vi "mining search for scenario.vi"(6 "User":T3, 7 "Header In":string, 8 "error in (no error)":errorcluster, 10 "GET (empty)":T1, 11 "Connection Refnum":T2) -> (0 "error out":errorcluster, 1 "Template Keys":T1, 2 "Template":string, 3 "Connection Refnum":T2, 5 "new Header":string)   [LabVIEW 2011]
uses:
  server/database/Users/User Record.ctl
  Addons/internet/utils/keyedarr.llb/Keyed Array.ctl
  SI.LIB/ODBC/SQL Controls/Connection Refnum.ctl
  Addons/internet/utils/strutil.llb/Case Matching.ctl
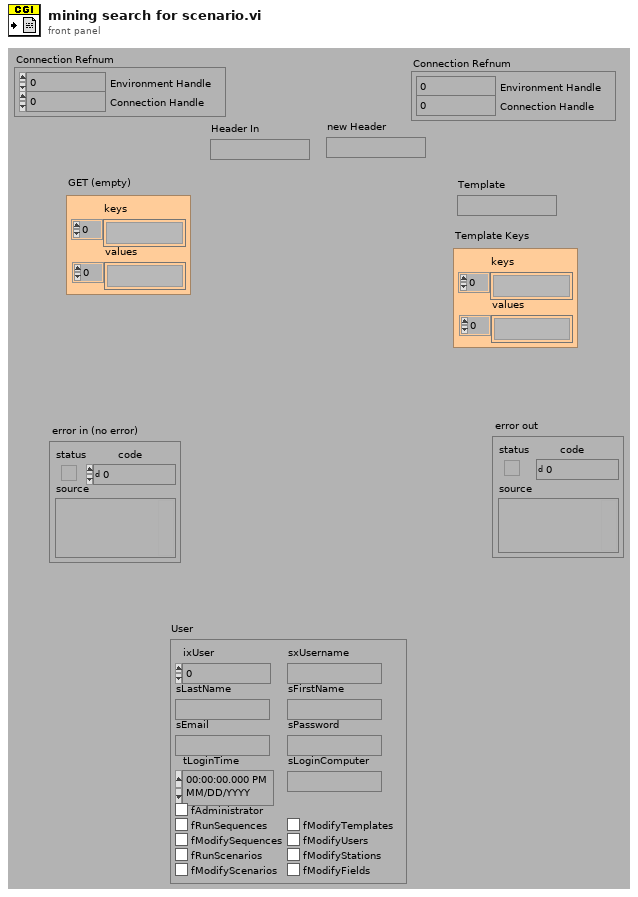
[diagram p1: front panel]
types:
  T1 = typedef "Keyed Array.ctl" = cluster{"keys":string[], "values":string[]}
  T2 = typedef "Connection Refnum.ctl" = cluster{"Environment Handle":i32, "Connection Handle":i32}
  T3 = typedef "User Record.ctl" = cluster{"ixUser":i32, "sxUsername":string, "sLastName":string, "sFirstName":string, "sEmail":string, "sPassword":string, "tLoginTime":timestamp, "sLoginComputer":string, "fAdministrator":bool, "fRunSequences":bool, "fModifySequences":bool, "fRunScenarios":bool, "fModifyScenarios":bool, "fModifyTemplates":bool, "fModifyUsers":bool, "fModifyStations":bool, "fModifyFields":bool}
  T4 = typedef "Case Matching.ctl" = enum16{"a != A", "a == A", "system"}
  T5 = typedef "Scenario Record.ctl" = cluster{"ixScenario":i32, "tCreated":timestamp, "tModified":timestamp, "sxUsername":string, "sModifiedBy":string, "sxScenarioId":string, "sDescription":string, "sLogic":string, "sResultFieldsCSV":string, "sTemplatesCSV":string, "fAutoRunReports":bool, "fSortByTemplates":bool, "fCombinePDF":bool, "Conditions":T6[]}
  T6 = typedef "Condition Record.ctl" = cluster{"iConditionIndex":i32, "sxFieldId":string, "nOperator":T7, "sMatchValue":string}
  T7 = typedef "Condition Operators.ctl" = enum16{"equal (=)", "not equal (\\u2260)", "less than (<)", "less than or equal (\\u2264)", "greater than (>)", "greater than or equal (\\u2265)", "contains", "does not contain"}
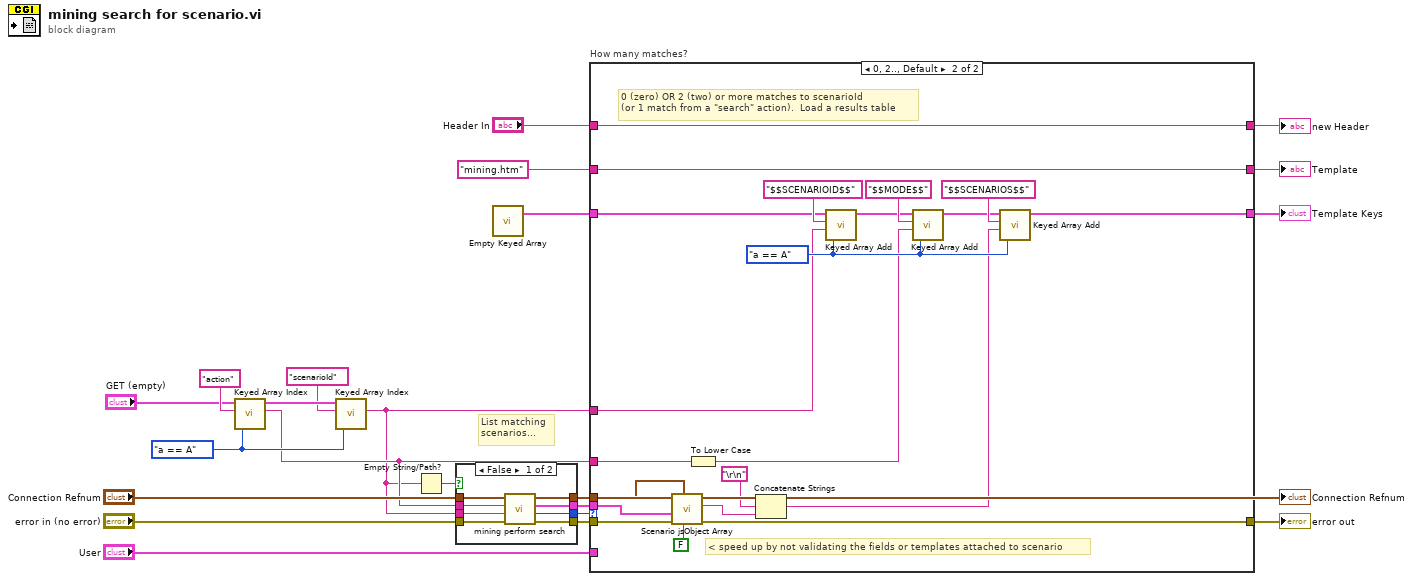
[diagram p0: block diagram]
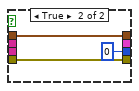
[diagram p2: hidden frame]
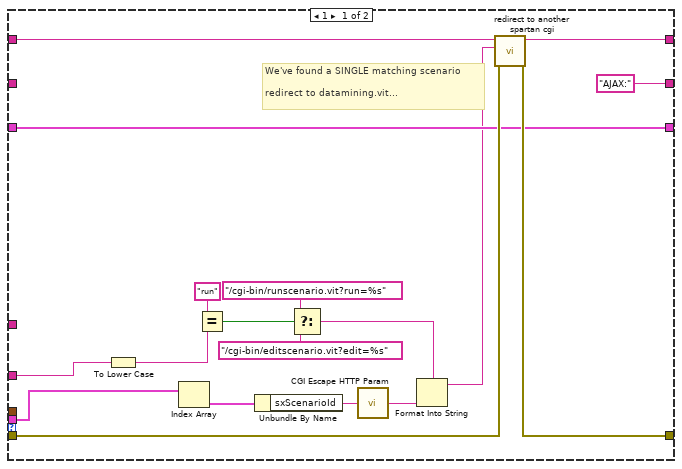
[diagram p3: hidden frame]
diagram:
  w8 = Case_Matching."a == A" ("case matching (sensitive)")
  # "List matching\nscenarios..."
  n1 = call "Keyed Array Index.vi"("case matching (sensitive)"=w8, "key"="action", "array in"="GET (empty)") -> ("value"=w7:string, "duplicate array"=w10:T1)  [unwired: 1 in, 2 out]
  n2 = call "Keyed Array Index.vi"("case matching (sensitive)"=w8, "key"="scenarioId", "array in"=w10) -> ("value"=w4:string)  [unwired: 1 in, 3 out]
  n3 = Empty String/Path?(string/path=w4) -> (empty?=w3:bool)
  n4 = case shown="False" w3 {
    tunnel: "error in (no error)" -> [w30 w32]
    tunnel: "Connection Refnum" -> [w29 w33]
    tunnel: [w28 w33] -> w2
    tunnel: [w27 _] -> w14
    tunnel: [w26 w32] -> w13
    tunnel: w7 -> [w25 _]
    tunnel: [w24 0 ("Matching Results")] -> w5
    tunnel: w4 -> [w23 _]
    frame False {
      n5 = call "mining perform search.vi"("error in (no error)"=w30, "sxScenarioId (\"\")"=w23, "Action (\"Search\")"=w25, "Connection Refnum"=w29) -> ("error out"=w26:errorcluster, "Matching Results"=w24:i32, "Results"=w27:T5[], "Connection Refnum"=w28:T2)  [unwired: 4 out]
    }
    frame True {
    }
  }
  "Connection Refnum" <- w2
  n6 = call "Empty Keyed Array.vi"() -> ("empty keyed array"=w19:T1)  [unwired: 3 out]
  n7 = case "How many matches?" shown="0, 2.., Default" w5 {
    tunnel: w4 -> [_ w55]
    tunnel: w14 -> [w41 w60]
    tunnel: "User" -> [_ _]
    tunnel: [w49 w65] -> w22
    tunnel: w19 -> [w49 w54]
    tunnel: w13 -> [w50 w62]
    tunnel: [w51 w61] -> w21
    tunnel: ["AJAX:" w70] -> w20
    tunnel: w7 -> [w44 w73]
    tunnel: [w46 w72] -> w17
    tunnel: "Header In" -> [w47 w72]
    tunnel: "mining.htm" ("Template (\"\")") -> [_ w70]
    tunnel: w2 -> [_ w53]
    frame 1 {
      # "We've found a SINGLE matching scenario\n\nredirect to datamining.vit..."
      n8 = To Lower Case(string=w44) -> (all lower case string=w42:string)
      n9 = Index Array(array=w41) -> (element=w40:T5)  [unwired: 1 in]
      n10 = Equal?(x="run" ("y"), y=w42) -> (x = y?=w39:bool)
      n11 = Unbundle By Name(w40) -> ("sxScenarioId"=w37:string)
      n12 = Select(t="/cgi-bin/runscenario.vit?run=%s" ("New URL (/cgi-bin/testing.vit)"), s=w39, f="/cgi-bin/editscenario.vit?edit=%s" ("New URL (/cgi-bin/testing.vit)")) -> (s? t:f=w34:string)
      n13 = call "CGI Escape HTTP Param.vi"("string"=w37) -> ("url-encoded string"=w38:string)
      n14 = Format Into String(format string=w34, w38) -> (resulting string=w45:string)  [unwired: 2 in, 1 out]
      n15 = call "redirect to another spartan cgi.vi"("error in (no error)"=w50, "New URL (/cgi-bin/testing.vit)"=w45, "Original Header In (to be replaced)"=w47) -> ("error out"=w51:errorcluster, "Redirection Header"=w46:string)  [unwired: 1 in, 6 out]
    }
    frame 0, 2.., Default {
      w66 = Case_Matching."a == A" ("case matching (sensitive)")
      # "< speed up by not validating the fields or templates attached to scenario"
      # "0 (zero) OR 2 (two) or more matches to scenarioId\n(or 1 match from a \"search\" action).  Load a results table"
      n16 = call "Scenario jsObject Array.vi"("Validate Fields/Templates? (t)"=FALSE, "Connection Refnum"=w53, "error in (no error)"=w62, "SCENARIOS (none)"=w60) -> ("error out"=w61:errorcluster, "Scenarios jsObject Array"=w58:string, "SCENARIOS jsObject Definition"=w59:string)  [unwired: 2 in, 3 out]
      n17 = To Lower Case(string=w73) -> (all lower case string=w63:string)
      n18 = Concatenate Strings(w59, "\r\n", w58) -> (w57:string)
      n19 = call "Keyed Array Add.vi"("case matching (sensitive)"=w66, "value"=w55, "key"="$$SCENARIOID$$", "array in"=w54) -> ("array out"=w64:T1)  [unwired: 3 out]
      n20 = call "Keyed Array Add.vi"("case matching (sensitive)"=w66, "value"=w63, "key"="$$MODE$$", "array in"=w64) -> ("array out"=w67:T1)  [unwired: 3 out]
      n21 = call "Keyed Array Add.vi"("case matching (sensitive)"=w66, "value"=w57, "key"="$$SCENARIOS$$", "array in"=w67) -> ("array out"=w65:T1)  [unwired: 3 out]
    }
  }
  "error out" <- w21
  "Template Keys" <- w22
  "Template" <- w20
  "new Header" <- w17
